vi "publisher tests Writer 11.vi"() -> ()   [LabVIEW 2018]
uses:
  publisher action.ctl
panel:
  out "Numeric":i32
  out "number":dbl
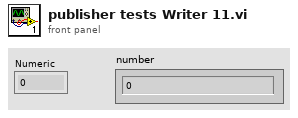
[diagram p1: front panel]
types:
  T1 = typedef "publisher action.ctl" = enum16{"set", "get", "init", "check"}
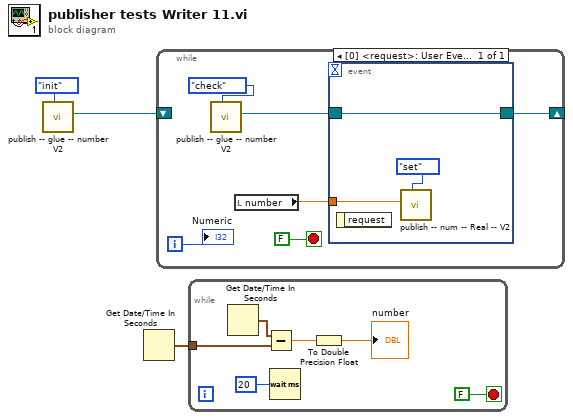
[diagram p0: block diagram]
diagram:
  n1 = call "publish -- glue -- number V2.vi"("publisher action"=publisher_action."init") -> ("Event Registration Refnum out"=w1:refnum<event-registration>)  [unwired: 9 in, 1 out]
  n2 = Get Date/Time In Seconds() -> (seconds since 1Jan1904=w3:timestamp)
  n3 = while {
    shift-right: [w6] -> _
    shift-left: w1 -> [_]
    i -> [w8]
    stop <- FALSE stop-if-true
    n4 = call "publish -- glue -- number V2.vi"("publisher action"=publisher_action."check") -> ("Event Registration Refnum out"=w5:refnum<event-registration>)  [unwired: 9 in, 1 out]
    n5 = local read "number"() -> (w7:dbl)
    n6 = event shown="[0] <request>: User Event" {
      selector: w5 -> [w12]
      dyn-events: [w12] -> w6
      timeout: _ -> [_]
      tunnel: w7 -> [w11]
      event User Event {
        n7 = event-data() -> ()  [unwired: 1 in, 1 out]
        n8 = call "publish -- num -- Real -- V2.vi"("publisher action"=publisher_action."set", "Numeric"=w11) -> ()  [unwired: 8 in, 2 out]
      }
    }
    "Numeric" <- w8
  }
  n9 = while {
    tunnel: w3 -> [w15]
    stop <- FALSE stop-if-true
    n10 = Get Date/Time In Seconds() -> (seconds since 1Jan1904=w17:timestamp)
    n11 = Subtract(x=w17, y=w15) -> (x-y=w18:dbl)
    n12 = Wait (ms)(milliseconds to wait=u32 20) -> ()  [unwired: 1 out]
    n13 = To Double Precision Float(number=w18) -> (double precision float=→"number":dbl)
  }
